vi "SPI.vi"(3 "Data to Write":u8[](array[numeric])=[0, 0, 0, 0, 0, 0, 0, 0, 0, 0] format="%x", 4 "Frames to Write":u8, 5 "SPI Config In":T1) -> (0 "Data Read":u8[](array[numeric]) format="%x", 1 "Frames Read":u8, 2 "SPI Config Out":T1)   [LabVIEW 2019]
uses:
  <vilib>/platform/TimedLoop/XDataNode/XDataNode.xnode
  <vilib>/Platform/TimedLoop/XDataNode/nitl_modes.ctl
  <vilib>/Platform/TimedLoop/XDataNode/XDNodeRunTimeDep.lvlib
  <vilib>/Platform/TimedLoop/XDataNode/wakeup.ctl
  <vilib>/Platform/TimedLoop/XDataNode/timing_clust.ctl
  <vilib>/eio/EIONode/EIONode.xnode
  <vilib>/rvi/eio/common/nirviEmuTemplateMethod_errors.vi
  SPI Config.ctl
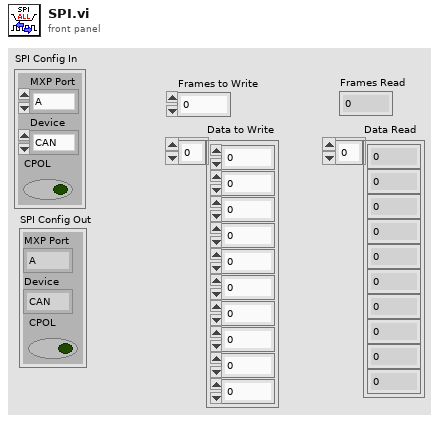
[diagram p1: front panel]
types:
  T1 = typedef "SPI Config.ctl" = cluster{"MXP Port":enum16{"A", "B"}, "Device":enum16{"CAN", "ENC", "IMU1", "IMU2"}, "CPOL":bool}
  T2 = typedef "XDNodeRunTimeDep.lvlib/timing_clust.ctl" = cluster{"Expected End [f-1]":u64, "Actual End [f-1]":u64, "Finished Late? [f-1]":bool, "Expected End [i-1]":u64, "Actual End [i-1]":u64, "Finished Late? [i-1]":bool, "Expected Start [i]":u64, "Actual Start [i]":u64, "Expected Start [f]":u64, "Actual Start [f]":u64, "Source Name":string, "Structure Name":string, "Period":i64, "Deadline":i64, "Offset":i64, "Start":i64, "Priority":i32, "Timeout":i32, "Mode":T3, "Wakeup Reason":T4, "Error":errorcluster, "Source Type":string, "Secondary Source Type":string, "Global End Time":u64, "Global Start Time":u64, "Frame Duration":u64, "Iteration Duration":u64, "Assigned CPU":i32, "I/O Scan Engine Mode":u32}
  T3 = typedef "XDNodeRunTimeDep.lvlib/nitl_modes.ctl" = enum32{"No Change", "Process missed periods, maintain original phase", "Discard missed periods, maintain original phase", "Process missed periods, ignore original phase", "Discard missed periods, ignore original phase"}
  T4 = typedef "XDNodeRunTimeDep.lvlib/wakeup.ctl" = enum32{"Normal", "Aborted", "Asynchronous wakeup", "Timing source error", "Timed loop error", "Timeout"}
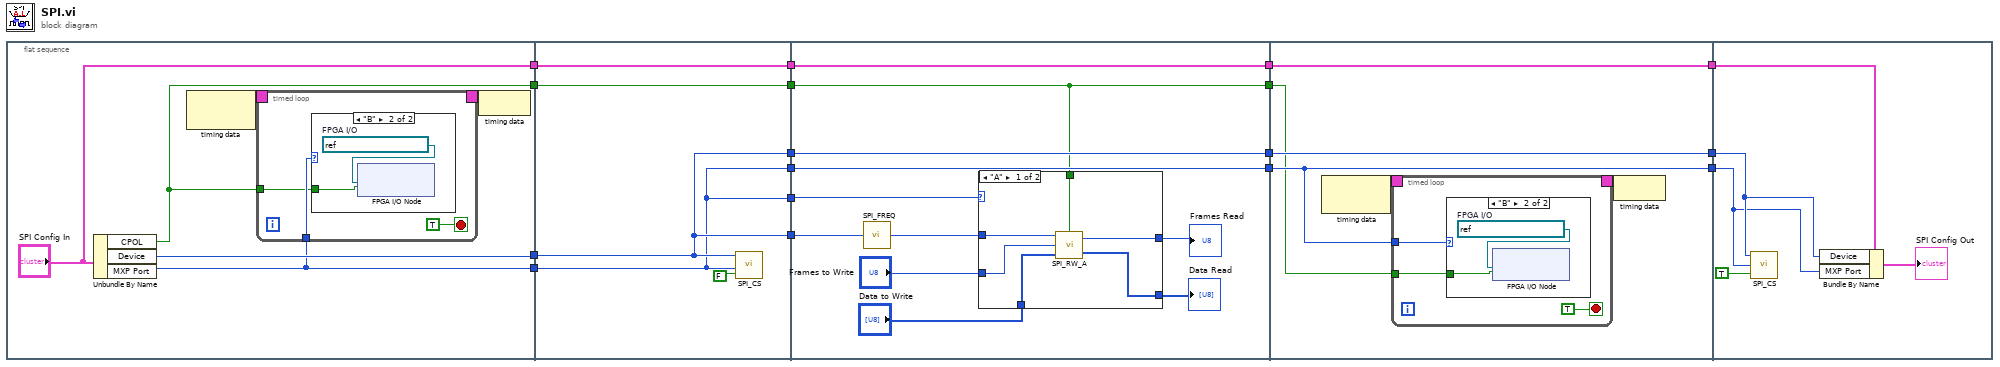
[diagram p0: block diagram]
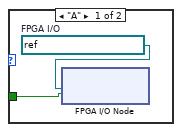
[diagram p2: hidden frame]
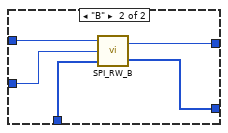
[diagram p3: hidden frame]
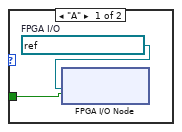
[diagram p4: hidden frame]
diagram:
  n1 = flat-sequence {
    tunnel: ["SPI Config In"] -> w12
    tunnel: [w22] -> w11
    tunnel: [w19] -> w10
    tunnel: [w18] -> w8
    tunnel: [w36] -> w17
    tunnel: [w36] -> w16
    tunnel: [w37] -> w15
    tunnel: [w38] -> w14
    tunnel: [w37] -> w13
    tunnel: w12 -> [w38]
    tunnel: w11 -> [w37]
    tunnel: w10 -> [w36]
    tunnel: [w35] -> w9
    tunnel: w8 -> [w35]
    tunnel: w17 -> [w46]
    tunnel: w16 -> [w45]
    tunnel: [w45] -> w7
    tunnel: [w44] -> w5
    tunnel: w15 -> [w44]
    tunnel: w14 -> [w43]
    tunnel: [w43] -> w3
    tunnel: w13 -> [w41]
    tunnel: w9 -> [w40]
    tunnel: [w40] -> w1
    tunnel: w7 -> [w63]
    tunnel: [w63] -> w6
    tunnel: w5 -> [w67]
    tunnel: [w67] -> w4
    tunnel: w3 -> [w66]
    tunnel: [w66] -> w2
    tunnel: w1 -> [w62]
    tunnel: w6 -> [w80]
    tunnel: w4 -> [w81]
    tunnel: w2 -> [w82]
    frame #0 {
      n2 = Unbundle By Name("SPI Config In") -> ("CPOL"=w18:bool, "Device"=w22:enum16{"CAN", "ENC", "IMU1", "IMU2"}, "MXP Port"=w19:enum16{"A", "B"})
      n3 = node-c288() -> (w21:T2)  [unwired: 1 in]
      n4 = timed-loop {
        timing: w21 -> [_]
        timing-out: [_] -> w20
        tunnel: w19 -> [w26]
        tunnel: w18 -> [w24]
        stop <- TRUE stop-if-true
        n5 = case shown="\"B\"" w26 {
          tunnel: w24 -> [w27 w29]
          frame "A" {
            w28 = refnum<k21> "ConnectorA/DIO5"  # FPGA I/O
            n6 = xnode "FPGA I/O Node"("I/O Item"=w27, "FPGA I/O In"=w28) -> ()  [unwired: 1 out]
          }
          frame "B" {
            w30 = refnum<k21> "ConnectorB/DIO5"  # FPGA I/O
            n7 = xnode "FPGA I/O Node"("I/O Item"=w29, "FPGA I/O In"=w30) -> ()  [unwired: 1 out]
          }
        }
      }
      n8 = node-c288(w20) -> ()
    }
    frame #1 {
      n9 = call "SPI_CS.vi"("Value"=FALSE, "MXP Port"=w36, "Device"=w37) -> ()
    }
    frame #2 {
      n10 = call "SPI_FREQ.vi"("Device"=w41) -> ("Frequency (kHz)"=w42:u16)
      n11 = case shown="\"A\"" w46 {
        tunnel: w42 -> [w56 w61]
        tunnel: "Frames to Write" -> [w55 w60]
        tunnel: "Data to Write" -> [w54 w59]
        tunnel: [w53 w58] -> w48
        tunnel: [w52 w57] -> w47
        tunnel: w40 -> [w51 _]
        frame "A" {
          n12 = call "SPI_RW_A.vi"("CPOL"=w51, "Data to Write"=w54, "Frames to Write"=w55, "SPI Frequency (KHz)"=w56) -> ("Data Read"=w52:u8[], "Frames Read"=w53:u8)
        }
        frame "B" {
          n13 = call "SPI_RW_B.vi"("Data to Write"=w59, "Frames to Write"=w60, "SPI Frequency (KHz)"=w61) -> ("Data Read"=w57:u8[], "Frames Read"=w58:u8)  [unwired: 1 in]
        }
      }
      "Frames Read" <- w48
      "Data Read" <- w47
    }
    frame #3 {
      n14 = node-c288() -> (w65:T2)  [unwired: 1 in]
      n15 = timed-loop {
        timing: w65 -> [_]
        timing-out: [_] -> w64
        tunnel: w63 -> [w70]
        tunnel: w62 -> [w68]
        stop <- TRUE stop-if-true
        n16 = case shown="\"B\"" w70 {
          tunnel: w68 -> [w71 w73]
          frame "A" {
            w72 = refnum<k21> "ConnectorA/DIO5"  # FPGA I/O
            n17 = xnode "FPGA I/O Node"("I/O Item"=w71, "FPGA I/O In"=w72) -> ()  [unwired: 1 out]
          }
          frame "B" {
            w74 = refnum<k21> "ConnectorB/DIO5"  # FPGA I/O
            n18 = xnode "FPGA I/O Node"("I/O Item"=w73, "FPGA I/O In"=w74) -> ()  [unwired: 1 out]
          }
        }
      }
      n19 = node-c288(w64) -> ()
    }
    frame #4 {
      n20 = call "SPI_CS.vi"("Value"=TRUE, "MXP Port"=w80, "Device"=w81) -> ()
      n21 = Bundle By Name(cluster=w82, "Device"=w81, "MXP Port"=w80) -> (→"SPI Config Out":T1)
    }
  }
